vi "Forklift Down.vi"(8 "Forklift Down Speed":dbl) -> ()   [LabVIEW 2014]
uses:
  <vilib>/Rock Robotics/WPI/Compressor/WPI_CompressorDevRef.ctl
  <vilib>/Rock Robotics/WPI/Solenoid/WPI_SolenoidValue.ctl
  _2015 Season/Mecanum Prototype v5/Mecanum Prototype v1/Robot Global Data.vi
  <vilib>/Rock Robotics/WPI/Solenoid/WPI_SolenoidSetEnum.vi
panel:
  in  "CompressorDevRef":T1
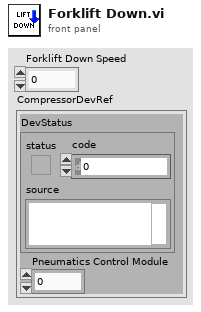
[diagram p1: front panel]
types:
  T1 = typedef "WPI_CompressorDevRef.ctl" = cluster{"DevStatus":errorcluster, "Pneumatics Control Module":u8}
  T2 = typedef "WPI_MotorControlDeviceRef.ctl" = cluster{"DeviceStatus":errorcluster, "Type":T3, "PWM":cluster{"Controller":T4, "PWM Channel":T5, "DeadBand":T6}, "CAN":cluster{"Device Number":u8, "Control Mode":T7, "Semaphore":T8, "Max Vout":dbl, "TalonSRX Control Mode":T9}, "Invert":bool, "TransformRef":T10, "InvTransformRef":T10}
  T3 = typedef "WPI_MotorControlType.ctl" = enum16{"PWM", "CAN", "CANTalonSRX"}
  T4 = typedef "FPGA_TypedefDigitalModule.ctl" = enum16{"Controller 1"}
  T5 = typedef "FPGA_DIOPWMChannel.ctl" = enum8{"PWM 0", "PWM 1", "PWM 2", "PWM 3", "PWM 4", "PWM 5", "PWM 6", "PWM 7", "PWM 8", "PWM 9", "PWM MXP 0", "PWM MXP 1", "PWM MXP 2", "PWM MXP 3", "PWM MXP 4", "PWM MXP 5", "PWM MXP 6", "PWM MXP 7", "PWM MXP 8", "PWM MXP 9", "Invalid"}
  T6 = typedef "WPI_PWMDeadband.ctl" = cluster{"Name":string, "maxPositivePwm":i32, "minPositivePwm":i32, "centerPwm":i32, "maxNegativePwm":i32, "minNegativePwm":i32, "angularRange":u16}
  T7 = typedef "WPI_CANJaguar_ControlMode.ctl" = enum8{"Percent VBus", "Current", "Speed", "Position", "Voltage"}
  T8 = typedef "Semaphore RefNum" = refnum<k1>
  T9 = typedef "WPI_CANTalonSRX_APIControlMode.ctl" = enum8{"Percent VBus", "Speed", "Position", "Slave", "Unchanged / Invalid"}
  T10 = typedef "WPI_PWMTransform_ConPane.ctl" = refnum<vi>
  T11 = typedef "WPI_SolenoidDevRef.ctl" = cluster{"DevStatus":errorcluster, "Pneumatics Control Module":u8, "Forward Solenoid Channel":T12, "Reverse Solenoid Channel":T12}
  T12 = typedef "WPI_SolenoidChannel.ctl" = enum8{"Solenoid 0", "Solenoid 1", "Solenoid 2", "Solenoid 3", "Solenoid 4", "Solenoid 5", "Solenoid 6", "Solenoid 7", "Invalid"}
  T13 = typedef "WPI_SolenoidValue.ctl" = enum16{"Off", "On", "Forward", "Reverse"}
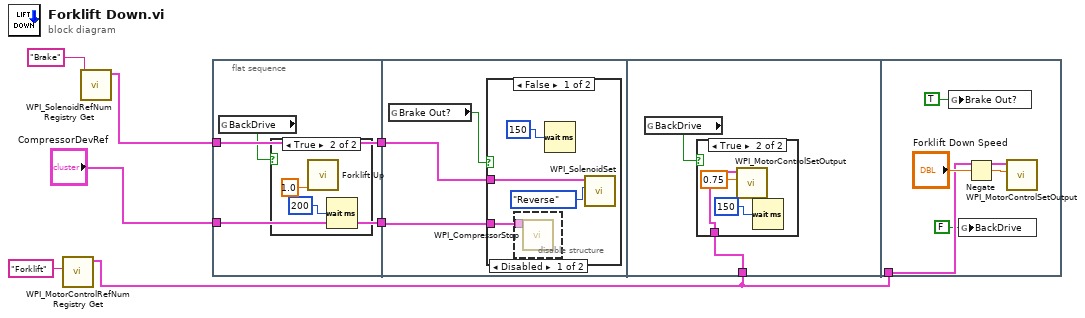
[diagram p0: block diagram]
diagram:
  n1 = call <vilib>:"WPI_MotorControlRefNum Registry Get.vi"("refnum name"="Forklift") -> ("MotorControlDevRef"=w3:T2)  [unwired: 9 in, 1 out]
  n2 = call <vilib>:"WPI_SolenoidRefNum Registry Get.vi"("refnum name"="Brake") -> ("SolenoidDevRef"=w4:T11)  [unwired: 9 in, 1 out]
  n3 = flat-sequence {
    tunnel: "CompressorDevRef" -> [w9]
    tunnel: w4 -> [w10]
    tunnel: [w10] -> w2
    tunnel: [w9] -> w1
    tunnel: w2 -> [w14]
    tunnel: w1 -> [w13]
    tunnel: w3 -> [w21]
    tunnel: w3 -> [w29]
    frame #0 {
      n4 = global read "Robot Global Data.vi" "BackDrive"() -> (w8:bool)
      n5 = case shown="True" w8 {
        frame False {
        }
        frame True {
          n6 = call "Forklift Up.vi"("Forklift Up Power"=1.0) -> ()  [unwired: 11 in]
          n7 = Wait (ms)(milliseconds to wait=u32 200) -> ()  [unwired: 1 out]
        }
      }
    }
    frame #1 {
      n8 = global read "Robot Global Data.vi" "Brake Out?"() -> (w15:bool)
      n9 = case shown="False" w15 {
        tunnel: w14 -> [w17 _]
        tunnel: w13 -> [w16 _]
        frame False {
          n10 = disable-structure shown="Disabled" {
            disable-tunnel: w16 -> [w20 _]
            frame Disabled {
              n11 = call <vilib>:"WPI_CompressorStop.vi"("CompressorDevRef"=w20) -> ()  [unwired: 9 in, 2 out]
            }
            frame Enabled {
            }
          }
          n12 = Wait (ms)(milliseconds to wait=u32 150) -> ()  [unwired: 1 out]
          n13 = call-poly <vilib>:"WPI_SolenoidSet.vi"("Value"=WPI_SolenoidValue."Reverse", "SolenoidDevRef"=w17) -> ()  [unwired: 8 in, 2 out]
        }
        frame True {
        }
      }
    }
    frame #2 {
      n14 = global read "Robot Global Data.vi" "BackDrive"() -> (w22:bool)
      n15 = case shown="True" w22 {
        tunnel: w21 -> [_ w24]
        frame False {
        }
        frame True {
          n16 = call <vilib>:"WPI_MotorControlSetOutput.vi"("Output"=0.75, "MotorControlDevRef"=w24) -> ()  [unwired: 7 in, 3 out]
          n17 = Wait (ms)(milliseconds to wait=u32 150) -> ()  [unwired: 1 out]
        }
      }
    }
    frame #3 {
      n18 = global write "Robot Global Data.vi" "Brake Out?"(TRUE ("Brake Out?")) -> ()
      n19 = global write "Robot Global Data.vi" "BackDrive"(FALSE ("BackDrive")) -> ()
      n20 = Negate(x="Forklift Down Speed") -> (-x=w28:dbl)
      n21 = call <vilib>:"WPI_MotorControlSetOutput.vi"("Output"=w28, "MotorControlDevRef"=w29) -> ()  [unwired: 7 in, 3 out]
    }
  }
